vi "cDAQ Reset.vi"(8 "error in":errorcluster, 11 "DAQmx Device":tag="BoardTestStand") -> (0 "error out":errorcluster)   [LabVIEW 2022 SP3]
doc: "This VI will perform a self test of the cDAQ device"
panel:
  in  "stop":bool
  out "Unsuccesful Attempts to connect":i32
  out "Instructional Message":string
  out "Loop Error?":errorcluster
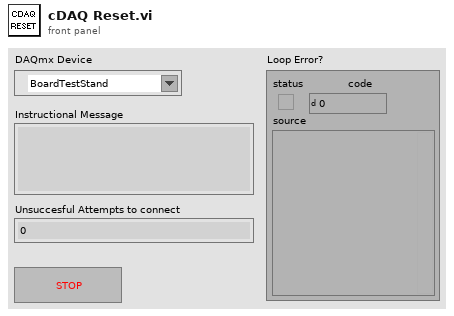
[diagram p1: front panel]
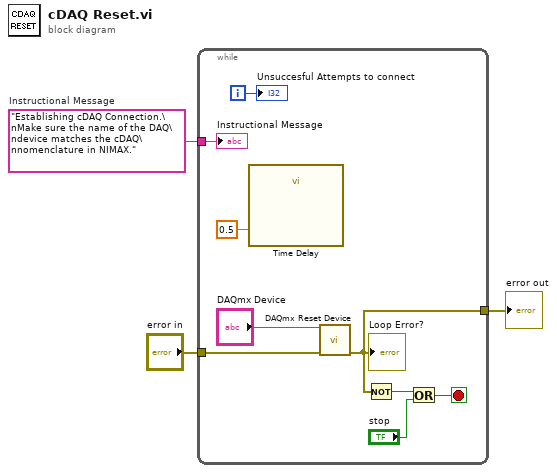
[diagram p0: block diagram]
diagram:
  w1 = "Establishing cDAQ Connection.\nMake sure the name of the DAQ\ndevice matches the cDAQ\nnomenclature in NIMAX."  # Instructional Message
  n1 = while {
    tunnel: "error in" -> [w12]
    tunnel: [w9] -> w2
    tunnel: w1 -> [w11]
    i -> [w10]
    stop <- w6 stop-if-true
    n2 = call "Time Delay"("Delay Time (s)"=0.5) -> ()  [unwired: 10 in, 1 out]
    n3 = call <vilib>:"DAQmx Reset Device.vi"("device in"="DAQmx Device", "error in"=w12) -> ("error out"=w9:errorcluster)  [unwired: 13 in]
    "Loop Error?" <- w9
    n4 = Not(x=w9) -> (.not. x?=w8:bool)
    n5 = Or(x=w8, y="stop") -> (x .or. y?=w6:bool)
    "Instructional Message" <- w11
    "Unsuccesful Attempts to connect" <- w10
  }
  "error out" <- w2
